vi "SQL Commands.vi"(8 "error in (no error)":errorcluster, 10 "connection reference":T1) -> (0 "error out":errorcluster, 2 "connection reference 2":T1)   [LabVIEW 2015]
uses:
  <vilib>/addons/database/Connection.llb/Conn ObjectReference.ctl
  <vilib>/addons/database/Connection.llb/Conn Execute.vi
  <vilib>/addons/database/NI_Database_API.lvlib
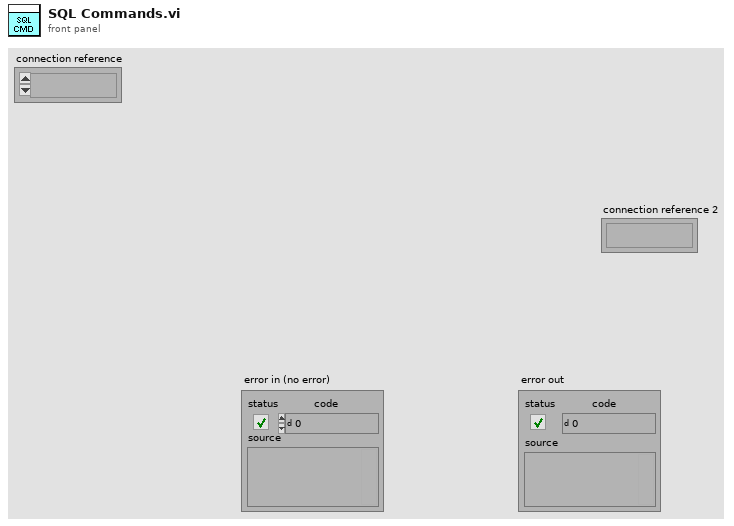
[diagram p1: front panel]
types:
  T1 = typedef "NI_Database_API.lvlib/Conn ObjectReference.ctl" = refnum<k1>
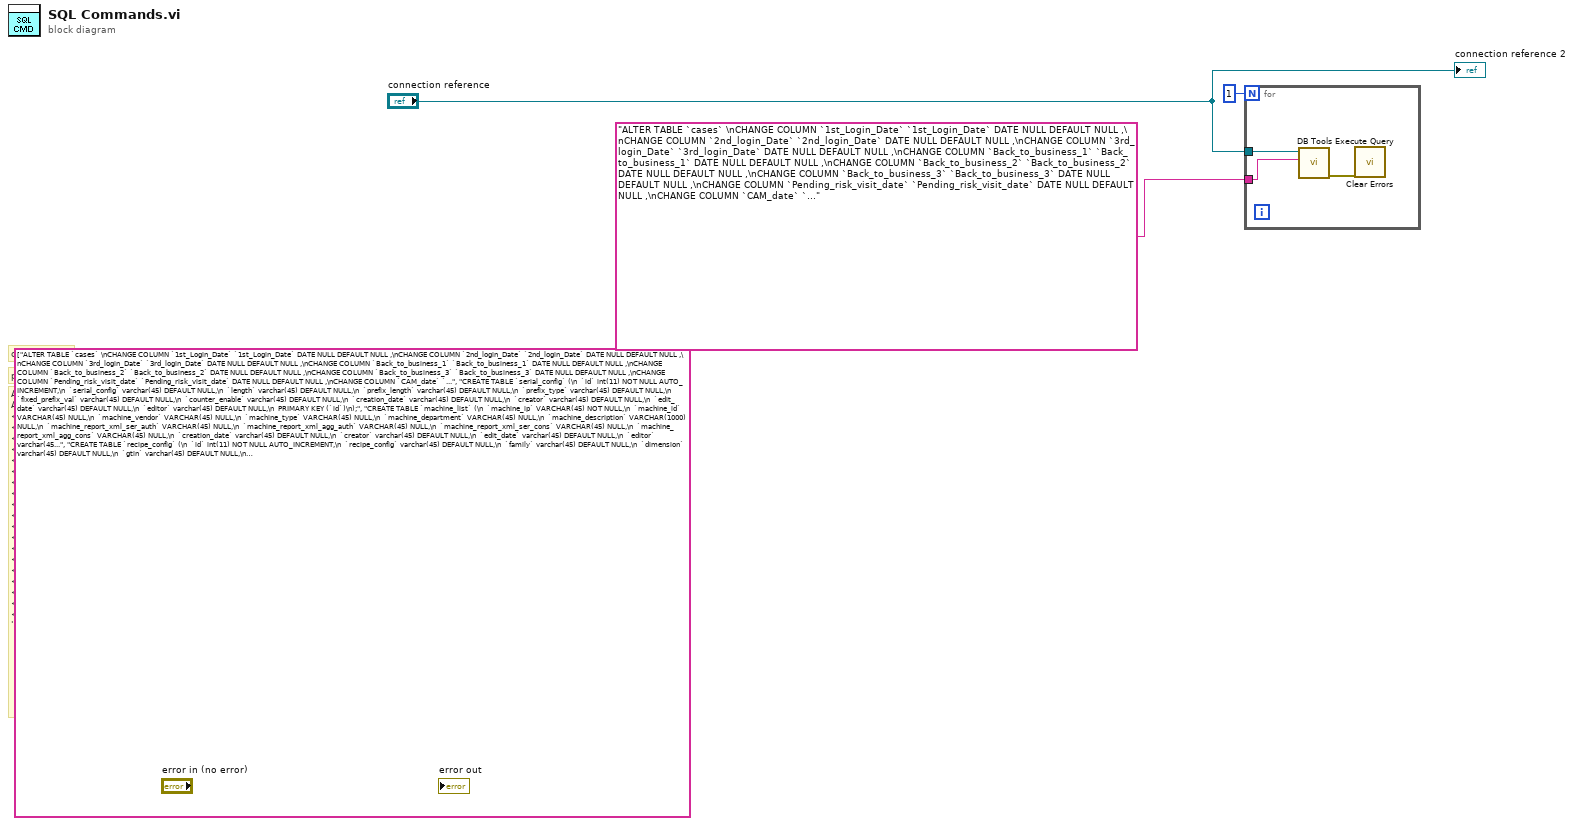
[diagram p0: block diagram]
diagram:
  (unwired) string[] ["ALTER TABLE `cases` \nCHANGE COLUMN `1st_Login_Date` `1st_Login_Date` DATE NULL DEFAULT NULL ,\nCHANGE COLUMN `2nd_login_Date` `2nd_login_Date` DATE NULL DEFAULT NULL ,\nCHANGE COLUMN `3rd_login_Date` `3rd_login_Date` DATE NULL DEFAULT NULL ,\nCHANGE COLUMN `Back_to_business_1` `Back_to_business_1` DATE NULL DEFAULT NULL ,\nCHANGE COLUMN `Back_to_business_2` `Back_to_business_2` DATE NULL DEFAULT NULL ,\nCHANGE COLUMN `Back_to_business_3` `Back_to_business_3` DATE NULL DEFAULT NULL ,\nCHANGE COLUMN `Pending_risk_visit_date` `Pending_risk_visit_date` DATE NULL DEFAULT NULL ,\nCHANGE COLUMN `CAM_date` `CAM_date` DATE NULL DEFAULT NULL ,\nCHANGE COLUMN `decline_date` `decline_date` DATE NULL DEFAULT NULL ,\nCHANGE COLUMN `CAD_submission_date` `CAD_submission_date` DATE NULL DEFAULT NULL ,\nCHANGE COLUMN `Stamped_date` `Stamped_date` DATE NULL DEFAULT NULL ,\nCHANGE COLUMN `Next_Review_date` `Next_Review_date` DATE NULL DEFAULT NULL ,\nCHANGE COLUMN `Business_Replay_date` `Business_Replay_date` DATE NULL DEFAULT NULL ;\n", "CREATE TABLE `serial_config` (\n  `id` int(11) NOT NULL AUTO_INCREMENT,\n  `serial_config` varchar(45) DEFAULT NULL,\n  `length` varchar(45) DEFAULT NULL,\n  `prefix_length` varchar(45) DEFAULT NULL,\n  `prefix_type` varchar(45) DEFAULT NULL,\n  `fixed_prefix_val` varchar(45) DEFAULT NULL,\n  `counter_enable` varchar(45) DEFAULT NULL,\n  `creation_date` varchar(45) DEFAULT NULL,\n  `creator` varchar(45) DEFAULT NULL,\n  `edit_date` varchar(45) DEFAULT NULL,\n  `editor` varchar(45) DEFAULT NULL,\n  PRIMARY KEY (`id`)\n);", "CREATE TABLE `machine_list` (\n  `machine_ip` VARCHAR(45) NOT NULL,\n  `machine_id` VARCHAR(45) NULL,\n  `machine_vendor` VARCHAR(45) NULL,\n  `machine_type` VARCHAR(45) NULL,\n  `machine_department` VARCHAR(45) NULL,\n  `machine_description` VARCHAR(1000) NULL,\n  `machine_report_xml_ser_auth` VARCHAR(45) NULL,\n  `machine_report_xml_agg_auth` VARCHAR(45) NULL,\n  `machine_report_xml_ser_cons` VARCHAR(45) NULL,\n  `machine_report_xml_agg_cons` VARCHAR(45) NULL,\n  `creation_date` varchar(45) DEFAULT NULL,\n  `creator` varchar(45) DEFAULT NULL,\n  `edit_date` varchar(45) DEFAULT NULL,\n  `editor` varchar(45) DEFAULT NULL,\n  PRIMARY KEY (`machine_ip`));\n", "CREATE TABLE `recipe_config` (\n  `id` int(11) NOT NULL AUTO_INCREMENT,\n  `recipe_config` varchar(45) DEFAULT NULL,\n  `family` varchar(45) DEFAULT NULL,\n  `dimension` varchar(45) DEFAULT NULL,\n  `gtin` varchar(45) DEFAULT NULL,\n  `agg_level` varchar(45) DEFAULT NULL,\n  `num_crtn_per_layer` varchar(45) DEFAULT NULL,\n  `creation_date` varchar(45) DEFAULT NULL,\n  `creator` varchar(45) DEFAULT NULL,\n  `edit_date` varchar(45) DEFAULT NULL,\n  `editor` varchar(45) DEFAULT NULL,\n  PRIMARY KEY (`id`)\n);", "CREATE TABLE `dep_list` (\n  `dep_name` VARCHAR(45) NOT NULL,\n  `creation_date` varchar(45) DEFAULT NULL,\n  `creator` varchar(45) DEFAULT NULL,\n  `edit_date` varchar(45) DEFAULT NULL,\n  `editor` varchar(45) DEFAULT NULL,\n  PRIMARY KEY (`dep_name`));\n", "ALTER TABLE `machine_list` \nADD COLUMN `xml_download_path` VARCHAR(45) NULL AFTER `machine_report_xml_agg_cons`,\nADD COLUMN `xml_upload_path` VARCHAR(45) NULL AFTER `xml_download_path`;\n", "ALTER TABLE `work_order` \nADD COLUMN `edit_date` VARCHAR(45) NULL AFTER `releaser`,\nADD COLUMN `editor` VARCHAR(45) NULL AFTER `edit_date`;\n", "CREATE TABLE `sscc_config` (\n  `sscc_config` VARCHAR(45) NOT NULL,\n  `extension_digit` VARCHAR(45) NOT NULL,\n  `prefix_length` VARCHAR(45) NOT NULL,\n  `prefix_value` VARCHAR(45) NOT NULL,\n  `serial_length` VARCHAR(45) NOT NULL,\n  `serial_type` VARCHAR(45) NOT NULL,\n  `creation_date` varchar(45) DEFAULT NULL,\n  `creator` varchar(45) DEFAULT NULL,\n  `edit_date` varchar(45) DEFAULT NULL,\n  `editor` varchar(45) DEFAULT NULL,\n  PRIMARY KEY (`sscc_config`));\n", "ALTER TABLE  `vision_config` \nADD COLUMN `layers_area_config` VARCHAR(1000) NULL DEFAULT '<Cluster>\r\n<Name>Layer Are Config</Name>\r\n<NumElts>6</NumElts>\r\n<DBL>\r\n<Name>Layer1 Area Min</Name>\r\n<Val>3000.00000000000000</Val>\r\n</DBL>\r\n<DBL>\r\n<Name>Layer1 Area Max</Name>\r\n<Val>7999.99999999999999</Val>\r\n</DBL>\r\n<DBL>\r\n<Name>Layer2 Area Min</Name>\r\n<Val>3000.00000000000000</Val>\r\n</DBL>\r\n<DBL>\r\n<Name>Layer2 Area Max</Name>\r\n<Val>7999.99999999999999</Val>\r\n</DBL>\r\n<DBL>\r\n<Name>Layer3 Area Min</Name>\r\n<Val>3000.00000000000000</Val>\r\n</DBL>\r\n<DBL>\r\n<Name>Layer3 Area Max</Name>\r\n<Val>7999.99999999999999</Val>\r\n</DBL>\r\n</Cluster>\r\n\r\n' AFTER `creator`;\n\n", "ALTER TABLE  `sscc_data` \nADD COLUMN `sscc_3` VARCHAR(45) DEFAULT '' AFTER `sscc_2`;", "ALTER TABLE  `sscc_data` \nADD COLUMN `sscc_2` VARCHAR(45) DEFAULT '' AFTER `sscc`;", "ALTER TABLE `work_order` \nADD COLUMN `l3_child_count` VARCHAR(45) NULL AFTER `agg_level`;", "ALTER TABLE `work_order` \nADD COLUMN `l4_child_count` VARCHAR(45) NULL AFTER `l3_child_count`;", "ALTER TABLE `itx_agg_mng`.`machine_list` \nADD COLUMN `sscc_id` VARCHAR(45) NULL DEFAULT NULL AFTER `xml_upload_path`;\n", "ALTER TABLE `itx_agg_mng`.`config` \nADD COLUMN `pallet_labler_ip` VARCHAR(45) NULL AFTER `Labler_IP`;\n", "ALTER TABLE `itx_agg_mng`.`config` \nADD COLUMN `shipper_scanner_port` VARCHAR(45) NULL AFTER `pallet_labler_ip`,\nADD COLUMN `pallet_scanner_port` VARCHAR(45) NULL AFTER `shipper_scanner_port`;\n"]
  # "ALTER TABLE `printverify` \nADD COLUMN `gs1_select` VARCHAR(400) NULL DEFAULT '<Cluster>\n<Name>Value</Name>\n<NumElts>4</NumElts>\n<Boolean>\n<Name>GTIN</Name>\n<Val>1</Val>\n</Boolean>\n<Boolean>\n<Name>BATCH</Name>\n<Val>1</Val>\n</Boolean>\n<Boolean>\n<Name>MFG</Name>\n<Val>0</Val>\n</Boolean>\n<Boolean>\n<Name>EXP</Name>\n<Val>1</Val>\n</Boolean>\n</Cluster>\n' ;"
  # "printverify"
  # "consc error"
  n1 = for {
    N: 1 -> [_]
    tunnel: "connection reference" -> [w7]
    tunnel: "ALTER TABLE `cases` \nCHANGE COLUMN `1st_Login_Date` `1st_Login_Date` DATE NULL DEFAULT NULL ,\nCHANGE COLUMN `2nd_login_Date` `2nd_login_Date` DATE NULL DEFAULT NULL ,\nCHANGE COLUMN `3rd_login_Date` `3rd_login_Date` DATE NULL DEFAULT NULL ,\nCHANGE COLUMN `Back_to_business_1` `Back_to_business_1` DATE NULL DEFAULT NULL ,\nCHANGE COLUMN `Back_to_business_2` `Back_to_business_2` DATE NULL DEFAULT NULL ,\nCHANGE COLUMN `Back_to_business_3` `Back_to_business_3` DATE NULL DEFAULT NULL ,\nCHANGE COLUMN `Pending_risk_visit_date` `Pending_risk_visit_date` DATE NULL DEFAULT NULL ,\nCHANGE COLUMN `CAM_date` `CAM_date` DATE NULL DEFAULT NULL ,\nCHANGE COLUMN `decline_date` `decline_date` DATE NULL DEFAULT NULL ,\nCHANGE COLUMN `CAD_submission_date` `CAD_submission_date` DATE NULL DEFAULT NULL ,\nCHANGE COLUMN `Stamped_date` `Stamped_date` DATE NULL DEFAULT NULL ,\nCHANGE COLUMN `Next_Review_date` `Next_Review_date` DATE NULL DEFAULT NULL ,\nCHANGE COLUMN `Business_Replay_date` `Business_Replay_date` DATE NULL DEFAULT NULL ;\n" -> [w5]
    n2 = call-poly <vilib>:"DB Tools Execute Query.vi"("SQL query"=w5, "connection reference"=w7) -> ("error out"=w6:errorcluster)  [unwired: 6 in, 1 out]
    n3 = call <vilib>:"Clear Errors.vi"("error in (no error)"=w6) -> ()  [unwired: 5 in, 2 out]
  }
  "connection reference 2" <- "connection reference"
  "error out" <- "error in (no error)"
